vi "Init DMM.vi"(1 "Timeout (ms)":i32=2000, 4 "DMM Reset":bool, 5 "DMM Control References Array":T1, 6 "error in":errorcluster, 7 "DMM Config on Startup":enum16{"PC->DMM", "DMM->PC"}(ring)=enum."DMM->PC", 8 "DMM Model":T3, 9 "DMM Address":refnum<visa-resource-name>="GPIB0::5::INSTR") -> (0 "error out":errorcluster, 2 "Instrument Name":string, 3 "VISA resource name out":refnum<visa-resource-name>)   [LabVIEW 2020]
uses:
  Typedefs/DMM Models Control.ctl
  Typedefs/DMM Control Variable References.ctl
  <instrlib>/Agilent 34405/Agilent 34405.lvlib
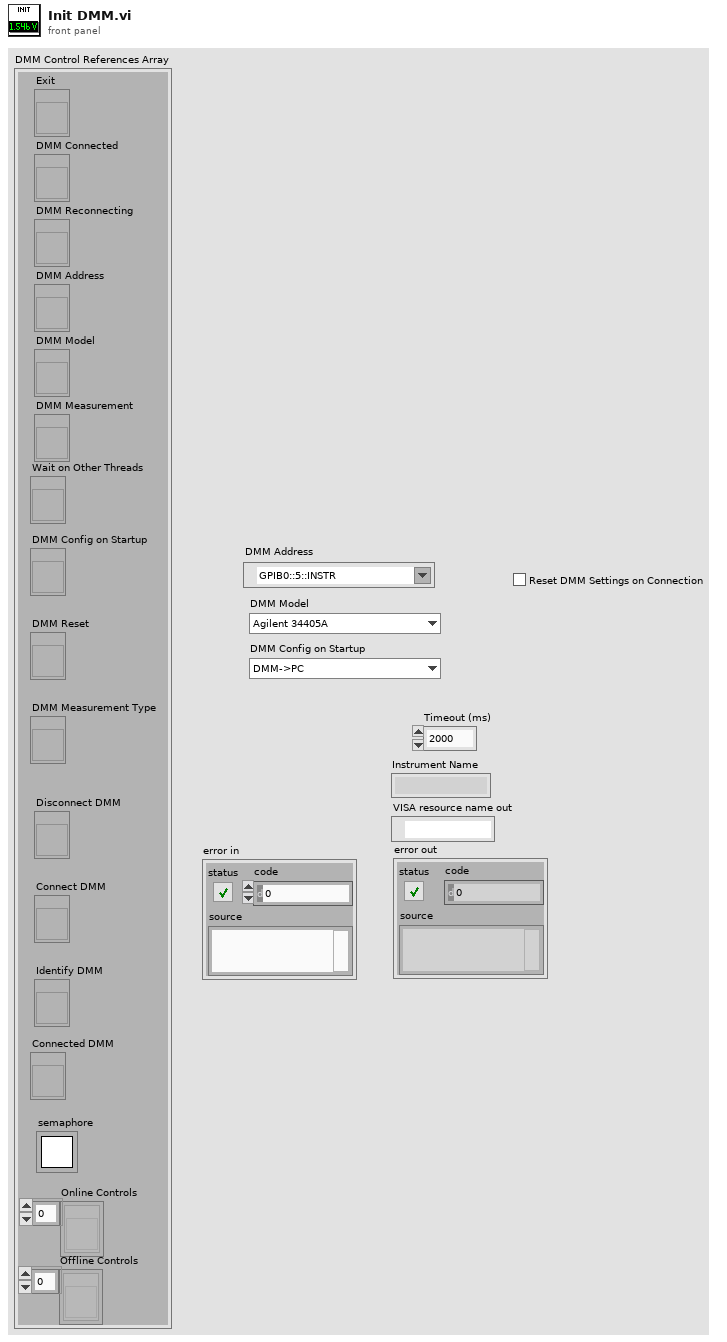
[diagram p1: front panel]
types:
  T1 = typedef "DMM Control Variable References.ctl" = cluster{"Exit":refnum<vi>, "DMM Connected":refnum<vi>, "DMM Reconnecting":refnum<vi>, "DMM Address":refnum<vi>, "DMM Model":refnum<vi>, "DMM Measurement":refnum<vi>, "Wait on Other Threads":refnum<vi>, "DMM Reset":refnum<vi>, "DMM Config on Startup":refnum<vi>, "DMM Measurement Type":refnum<vi>, "Disconnect DMM":refnum<vi>, "Connect DMM":refnum<vi>, "Identify DMM":refnum<vi>, "Connected DMM":refnum<vi>, "semaphore":T2, "Online Controls":refnum<vi>[], "Offline Controls":refnum<vi>[]}
  T2 = typedef "Semaphore RefNum" = refnum<k1>
  T3 = typedef "DMM Models Control.ctl" = enum16{"Agilent 34405A"}
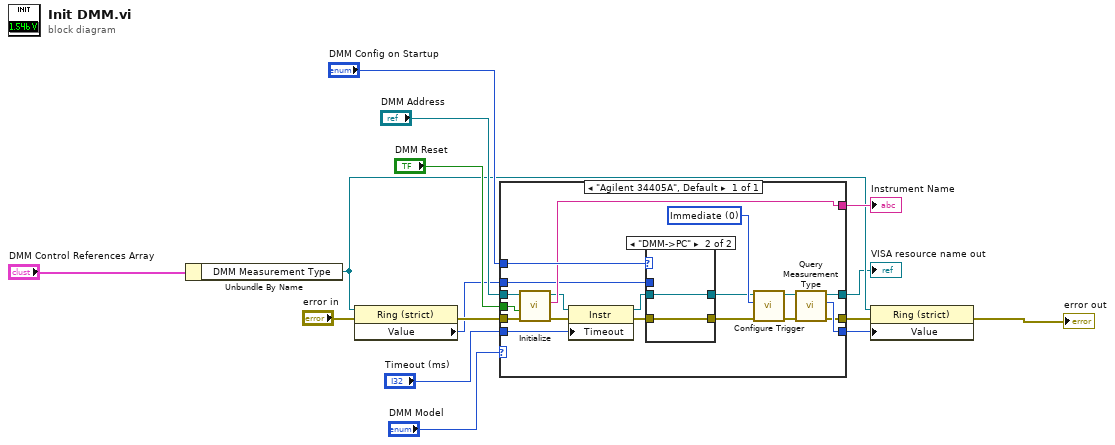
[diagram p0: block diagram]
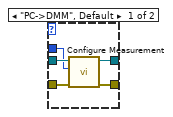
[diagram p2: hidden frame]
diagram:
  n1 = Unbundle By Name("DMM Control References Array") -> ("DMM Measurement Type"=w5:refnum<vi>)
  n2 = property class="Ring (strict)"(reference=w5, error in="error in") -> (error out=w8:errorcluster, "Value"=w7:i32)  [unwired: 1 out]
  n3 = case shown="\"Agilent 34405A\", Default" "DMM Model" {
    tunnel: "DMM Address" -> [w34]
    tunnel: "DMM Reset" -> [w33]
    tunnel: "DMM Config on Startup" -> [w31]
    tunnel: [w30] -> w12
    tunnel: "Timeout (ms)" -> [w25]
    tunnel: w8 -> [w24]
    tunnel: w7 -> [w23]
    tunnel: [w18] -> w6
    tunnel: [w17] -> w4
    tunnel: [w16] -> w3
    frame "Agilent 34405A", Default {
      w32 = 0 items=["Immediate", "Software (Bus)"] ("Trigger Source (0: Immediate)")
      n4 = call <instrlib>:"Initialize.vi"("error in (no error)"=w24, "Reset (True)"=w33, "VISA resource name"=w34) -> ("error out"=w29:errorcluster, "Instrument Name"=w30:string, "VISA resource name out"=w28:refnum<visa-resource-name>)  [unwired: 1 in, 5 out]
      n5 = property class="Instr"(reference=w28, error in=w29, "Timeout"=w25) -> (reference out=w27:refnum<visa-resource-name>, error out=w26:errorcluster)
      n6 = case shown="\"DMM->PC\"" w31 {
        tunnel: w26 -> [w35 w40]
        tunnel: w27 -> [w39 w41]
        tunnel: [w38 w41] -> w22
        tunnel: [w37 w40] -> w21
        tunnel: w23 -> [w36 _]
        frame "PC->DMM", Default {
          n7 = call <instrlib>:"Configure Measurement.vi"("error in (no error)"=w35, "Function (0: DC Volts)"=w36, "VISA resource name"=w39) -> ("error out"=w37:errorcluster, "VISA resource name out"=w38:refnum<visa-resource-name>)  [unwired: 7 in]
        }
        frame "DMM->PC" {
        }
      }
      n8 = call <instrlib>:"Configure Trigger.vi"("error in (no error)"=w21, "Trigger Source (0: Immediate)"=w32, "VISA resource name"=w22) -> ("error out"=w19:errorcluster, "VISA resource name out"=w20:refnum<visa-resource-name>)  [unwired: 7 out]
      n9 = call <instrlib>:"Query Measurement Type.vi"("error in (no error)"=w19, "VISA resource name"=w20) -> ("error out"=w17:errorcluster, "Measurement Type"=w18:u16, "VISA resource name out"=w16:refnum<visa-resource-name>)  [unwired: 7 in]
    }
  }
  "VISA resource name out" <- w3
  "Instrument Name" <- w12
  n10 = property class="Ring (strict)"(reference=w5, error in=w4, "Value"=w6) -> (error out=→"error out":errorcluster)  [unwired: 1 out]
